vi "setMicroscopeParameters.vi"(0 "Microscope in":refnum<class "Microscope.lvclass">, 5 "Scan Parameters":T2={"x pixels"=256, "x voltage min"=-2.0, "x voltage max"=2.0, "y voltage min"=256.0, "y voltage max"=-2.0, "fill frac"=2.0, "Zoom"=1.0, "BiDi"=FALSE, "scan rate (ms/line)"=2.0} {"Zoom" min=0.0 max=1.0 step=1.0; "fill frac" format="%0.2p"; "y voltage max" format="%0.2p"; "x voltage max" format="%0.2p"; "x voltage min" format="%0.2p"}, 7 "Hardware Settings":T1={"Galvo Channels"="Dev1/ao0:1", "Detector Channels"="Dev1/ai0:2", "Galvo Trigger"="/Dev1/ai/StartTrigger", "Shutter Lines"=["Dev1/port0/line7"], "Max Acquisition Rate"=5000000.0, "Recommended Acquisition Rate"=5000000.0, "Galvo Write Rate"=2500000.0, "Max Timebase Frequency (Hz)"=20000000.0, "MCC Shutter Lines"=[], "Detector Task"="", "Shutter Tasks"=[], "Galvo Task"="", "Digital Image Multiplier"=[100.0, 100.0, -100.0]} {"Max Acquisition Rate" min=0.0 max=5000000.0 step=100000.0}, 9 "Stage Acquire Parameters":T3={"Scan Mode"=enum."Continuous", "Start position mm"=115.0, "End position mm"=112.0, "Velocity um/sec (continuous)"=0.0, "Step size microns (discrete)"=2.0, "Frames to grab (grab)"=0}, 11 "error in (no error)":errorcluster) -> (4 "Microscope out":refnum<class "Microscope.lvclass">, 15 "error out":errorcluster)   [LabVIEW 2012, in "Microscope.lvclass"]
uses:
  classes/Microscope.lvclass
  typedefs/Stage Parameters.ctl
  typedefs/ScanMode.ctl
  typedefs/Scan Parameters.ctl
  typedefs/HWsettings.ctl
  classes/Microscope.lvclass/Microscope.ctl
  variables/GlobalUI.vi
  RotationProgram/Global/RotationGlobal.vi
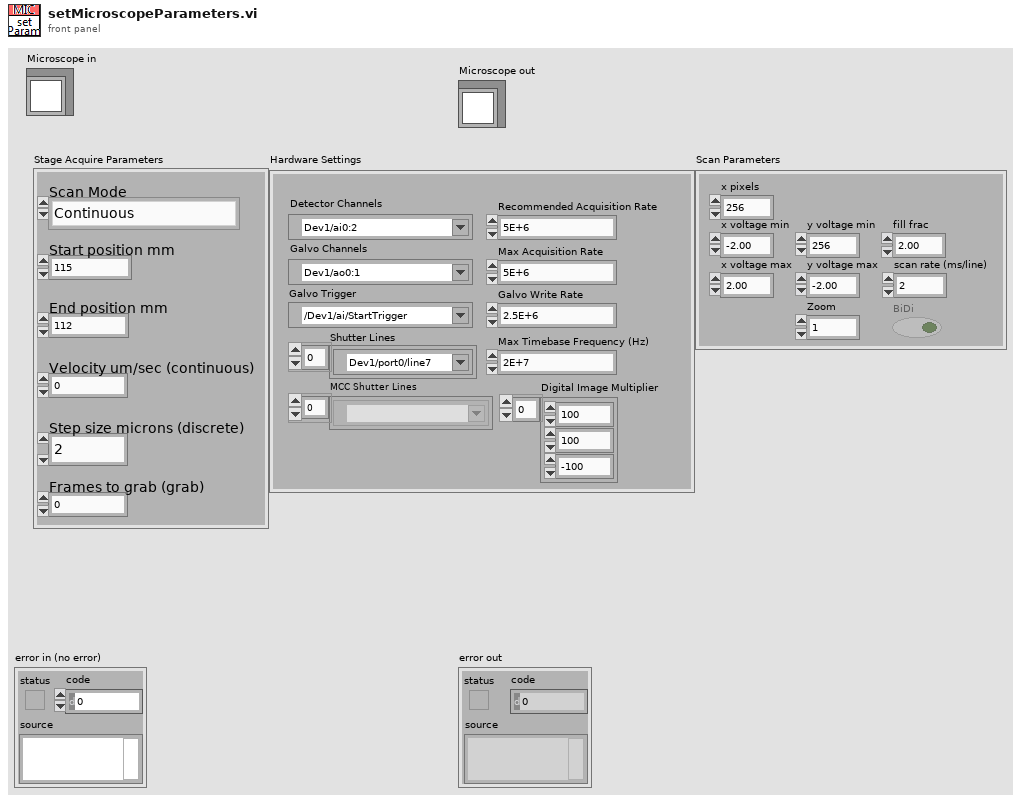
[diagram p1: front panel]
types:
  T1 = typedef "HWsettings.ctl" = cluster{"Galvo Channels":tag, "Detector Channels":tag, "Galvo Trigger":tag, "Shutter Lines":tag[], "Max Acquisition Rate":dbl, "Recommended Acquisition Rate":dbl, "Galvo Write Rate":dbl, "Max Timebase Frequency (Hz)":dbl, "MCC Shutter Lines":refnum<k21>[], "Detector Task":refnum<k21>, "Shutter Tasks":refnum<k21>[], "Galvo Task":refnum<k21>, "Digital Image Multiplier":dbl[]}
  T2 = typedef "Scan Parameters.ctl" = cluster{"x pixels":i32, "x voltage min":dbl, "x voltage max":dbl, "y voltage min":dbl, "y voltage max":dbl, "fill frac":dbl, "Zoom":dbl, "BiDi":bool, "scan rate (ms/line)":dbl}
  T3 = typedef "Stage Parameters.ctl" = cluster{"Scan Mode":T4, "Start position mm":dbl, "End position mm":dbl, "Velocity um/sec (continuous)":dbl, "Step size microns (discrete)":dbl, "Frames to grab (grab)":i32}
  T4 = typedef "ScanMode.ctl" = enum16{"None", "Continuous", "Point Scan (CH3 cursor)", "Point Scan Move (CH3 cursor)", "Grab", "Grab Move Stage", "Grab Move Z-stage", "Cont. Move Z-stage", "Spec Move Stage", "Spec Move Cont", "Surf Calib"}
  T5 = typedef "Scan Type.ctl" = enum16{"None", "Point", "Full Image Continuous", "Full Image Grab"}
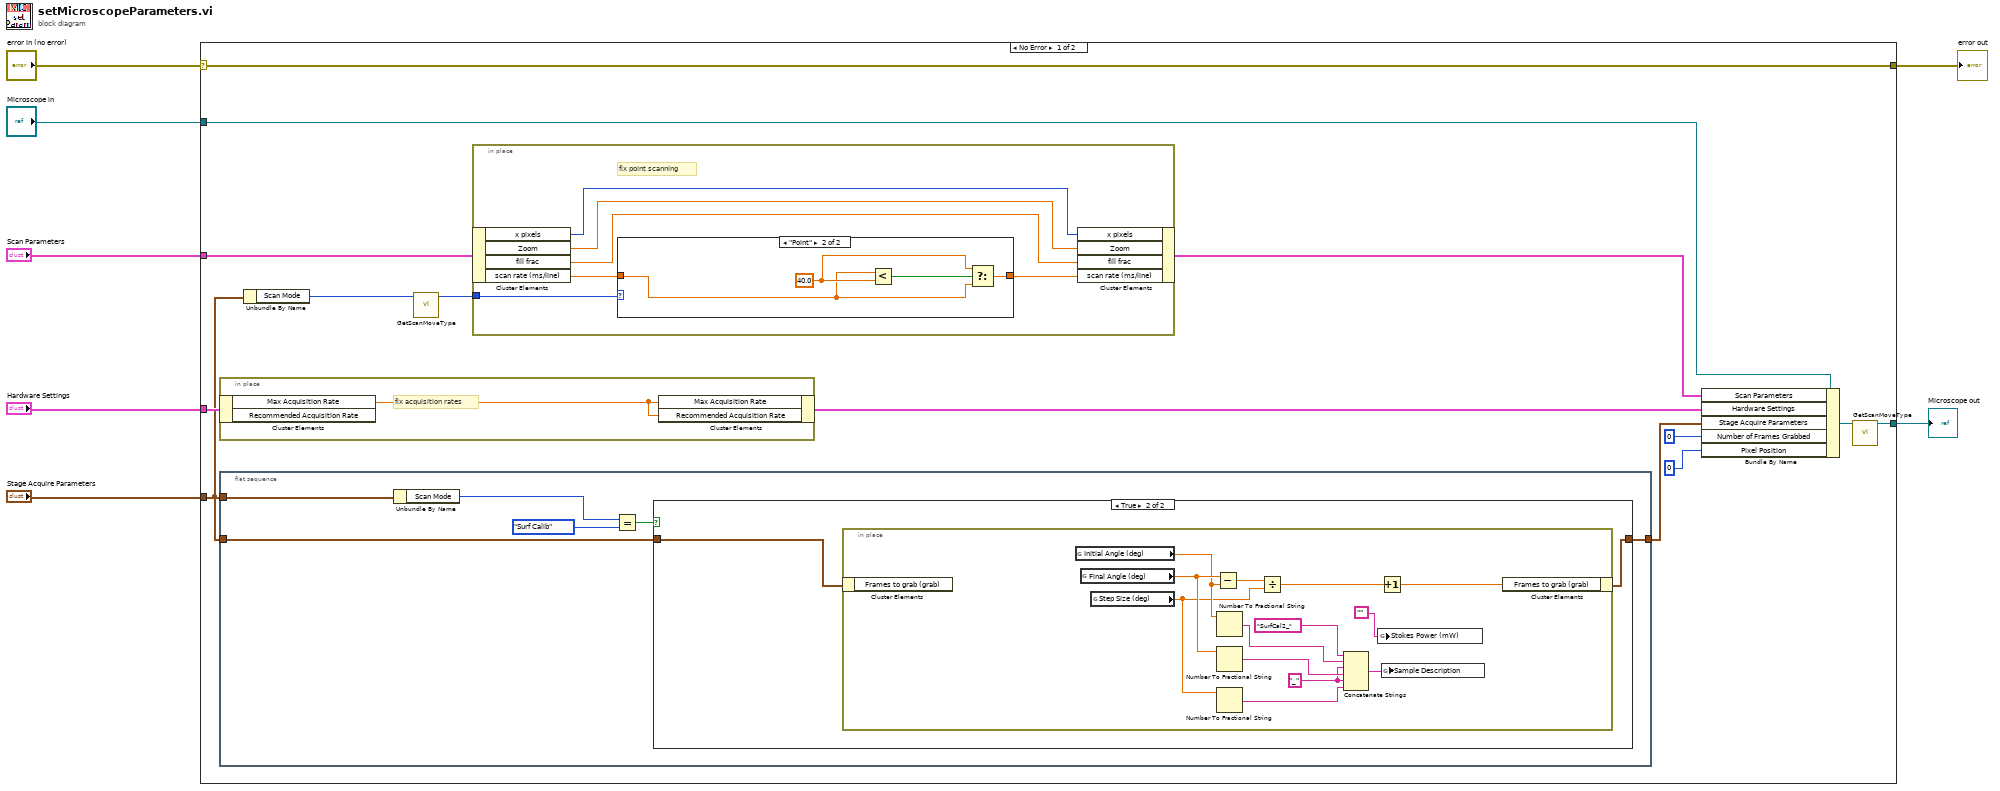
[diagram p0: block diagram]
diagram:
  n1 = case shown="No Error" "error in (no error)" {
    selector: "error in (no error)" -> [w21 w57]
    tunnel: [w21 w57] -> w6
    tunnel: [w11 w56] -> w4
    tunnel: "Microscope in" -> [w13 w56]
    tunnel: "Scan Parameters" -> [w16 _]
    tunnel: "Stage Acquire Parameters" -> [w9 _]
    tunnel: "Hardware Settings" -> [w20 _]
    frame No Error {
      n2 = in-place {
        # "fix acquisition rates"
        n3 = in-place-cluster #1(w20) -> ("Max Acquisition Rate"=w55:dbl)  [unwired: 1 out]
        n4 = in-place-cluster #1("Max Acquisition Rate"=w55, "Recommended Acquisition Rate"=w55) -> (w19:T1)
      }
      n5 = flat-sequence {
        tunnel: w9 -> [w27]
        tunnel: w9 -> [w24]
        tunnel: [w22] -> w8
        frame #0 {
          n6 = Unbundle By Name(w27) -> ("Scan Mode"=w26:T4)
          n7 = Equal?(x=w26, y=ScanMode."Surf Calib") -> (x = y?=w23:bool)
          n8 = case shown="True" w23 {
            tunnel: w24 -> [w28 w30]
            tunnel: [w28 w29] -> w22
            frame False {
            }
            frame True {
              n9 = in-place {
                w34 = "_" ("string")
                n10 = in-place-cluster #2(w30) -> ()  [unwired: 1 out]
                n11 = global read "RotationGlobal.vi" "Initial Angle (deg)"() -> (w39:dbl)
                n12 = global read "RotationGlobal.vi" "Final Angle (deg)"() -> (w40:dbl)
                n13 = global read "RotationGlobal.vi" "Step Size (deg)"() -> (w38:dbl)
                n14 = Subtract(x=w40, y=w39) -> (x-y=w43:dbl)
                n15 = Number To Fractional String(number=w39) -> (F-format string=w36:string)  [unwired: 3 in]
                n16 = Number To Fractional String(number=w40) -> (F-format string=w35:string)  [unwired: 3 in]
                n17 = Number To Fractional String(number=w38) -> (F-format string=w33:string)  [unwired: 3 in]
                n18 = Divide(x=w43, y=w38) -> (x/y=w42:dbl)
                n19 = Concatenate Strings("SurfCal2_" ("Sample Description"), w36, w34, w35, w34, w33) -> (w32:string)
                n20 = global write "GlobalUI.vi" "Stokes Power (mW)"("") -> ()
                n21 = Increment(x=w42) -> (x+1=w41:dbl)
                n22 = global write "GlobalUI.vi" "Sample Description"(w32) -> ()
                n23 = in-place-cluster #2("Frames to grab (grab)"=w41) -> (w29:T3)
              }
            }
          }
        }
      }
      n24 = Unbundle By Name(w9) -> ("Scan Mode"=w15:T4)
      n25 = call "GetScanMoveType.vi"("Scan Mode"=w15) -> ("Scan Type"=w14:T5)  [unwired: 8 in, 2 out]
      n26 = in-place {
        in-place-border: w14 -> [w44]
        # "fix point scanning"
        n27 = in-place-cluster #3(w16) -> ("x pixels"=w49:i32, "Zoom"=w48:dbl, "fill frac"=w47:dbl, "scan rate (ms/line)"=w46:dbl)
        n28 = case shown="\"Point\"" w44 {
          tunnel: w46 -> [w50 w52]
          tunnel: [w50 w51] -> w45
          frame "None", Default {
          }
          frame "Point" {
            w53 = 40.0 ("y")
            n29 = Less?(x=w52, y=w53) -> (x < y?=w54:bool)
            n30 = Select(t=w53, s=w54, f=w52) -> (s? t:f=w51:dbl)
          }
        }
        n31 = in-place-cluster #3("x pixels"=w49, "Zoom"=w48, "fill frac"=w47, "scan rate (ms/line)"=w45) -> (w10:T2)
      }
      n32 = Bundle By Name(cluster=w13, "Scan Parameters"=w10, "Hardware Settings"=w19, "Stage Acquire Parameters"=w8, "Number of Frames Grabbed"=0, "Pixel Position"=0) -> (w12:refnum<class "Microscope.lvclass">)
      n33 = call "GetScanMoveType.vi"("Microscope in"=w12) -> ("Microscope out"=w11:refnum<class "Microscope.lvclass">)  [unwired: 9 in, 1 out]
    }
    frame Error {
    }
  }
  "error out" <- w6
  "Microscope out" <- w4
